vi "Exec-tempalate-test.vi"() -> ()   [LabVIEW 2021]
uses:
  Controls/Command_cluster.ctl
  Controls/Command_Enum.ctl
panel:
  in  "file (use dialog)":path
  out "index of element":i32
  out "Command":string
  in  "stop":bool
  out "1D Array":T1[](array[typedef])
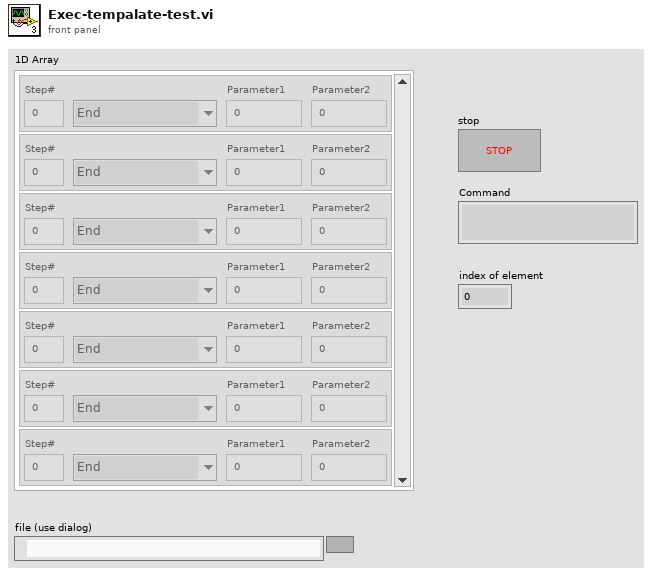
[diagram p1: front panel]
types:
  T1 = typedef "Command_cluster.ctl" = cluster{"Step#":dbl, "Commands":T2, "Parameter1":dbl, "Parameter2":dbl}
  T2 = typedef "Command_Enum.ctl" = enum16{"End", "Home All", "X Home", "Y Home", "X Move Rel", "X Move Abs", "Y Move Rel", "Y Move Abs", "Repeat", "Go To"}
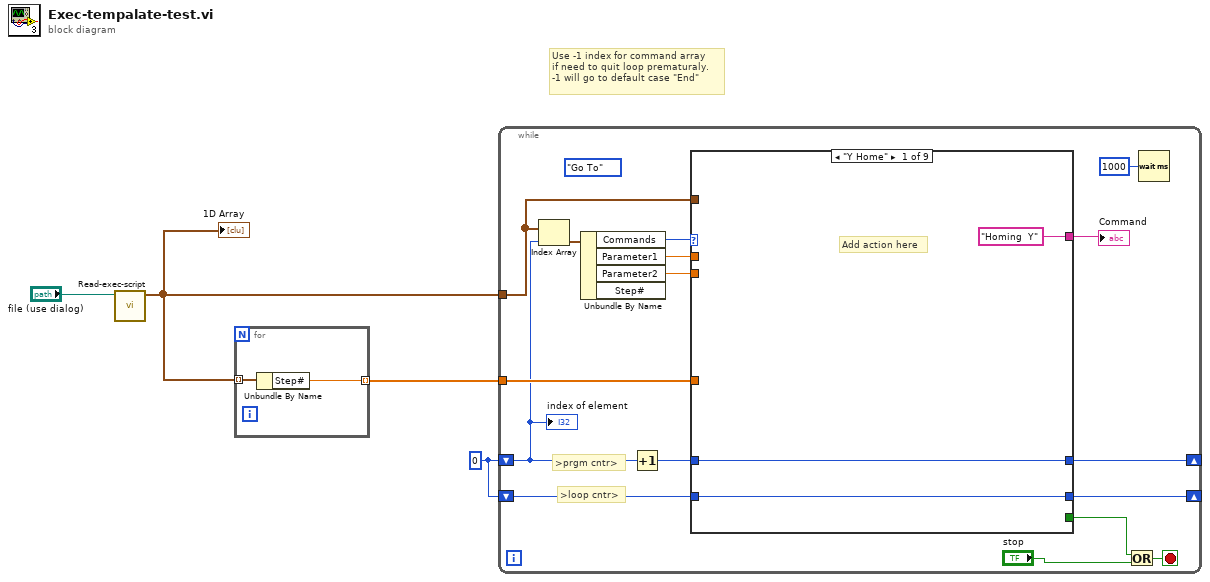
[diagram p0: block diagram]
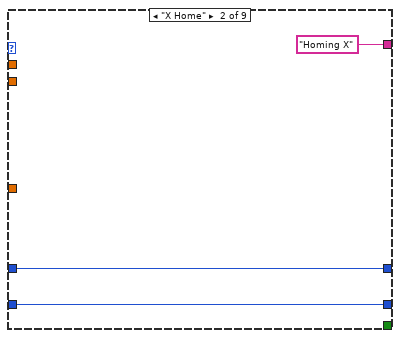
[diagram p2: hidden frame]
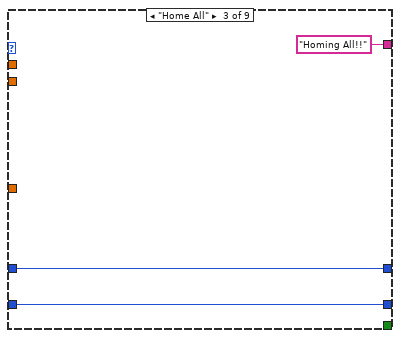
[diagram p3: hidden frame]
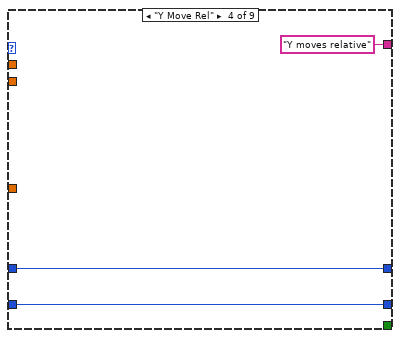
[diagram p4: hidden frame]
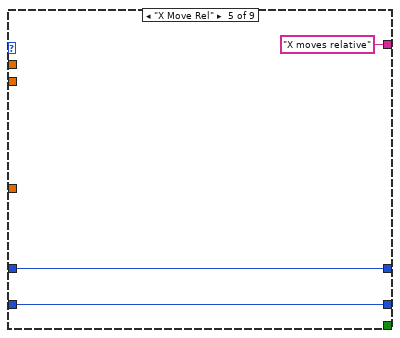
[diagram p5: hidden frame]
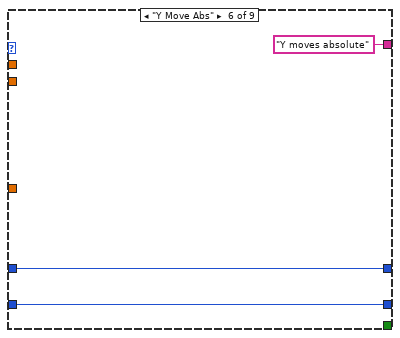
[diagram p6: hidden frame]
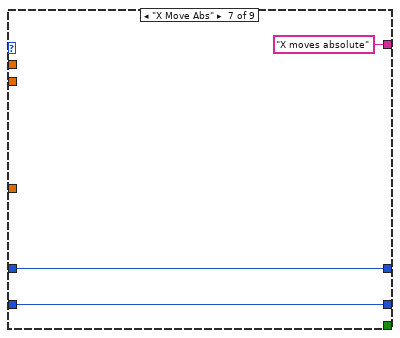
[diagram p7: hidden frame]
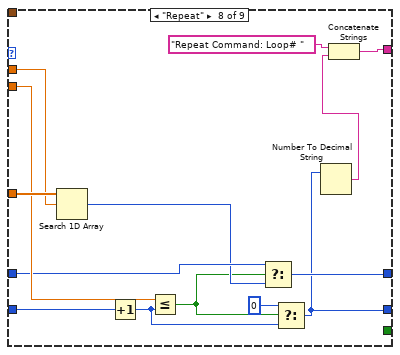
[diagram p8: hidden frame]
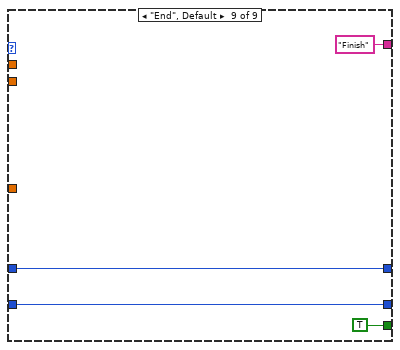
[diagram p9: hidden frame]
diagram:
  w3 = 0
  # "Use -1 index for command array\nif need to quit loop prematuraly.\n-1 will go to default case \"End\""
  n1 = call "Read-exec-script.vi"("file (use dialog)"="file (use dialog)") -> ("Commands"=w2:T1[])  [unwired: 9 in, 1 out]
  "1D Array" <- w2
  n2 = for {
    tunnel: w2 -> [w6] mode=indexing
    tunnel: [w5] -> w4 mode=indexing
    n3 = Unbundle By Name(w6) -> ("Step#"=w5:dbl)
  }
  n4 = while {
    tunnel: w2 -> [w17]
    tunnel: w4 -> [w18]
    shift-right: [w15] -> _
    shift-left: w3 -> [w8]
    shift-right: [w12] -> _
    shift-left: w3 -> [w16]
    stop <- w11 stop-if-true
    (unwired) Command_Enum."Go To" ("Commands")
    # ">loop cntr>"
    # ">prgm cntr>"
    n5 = Index Array(array=w17, index=w8) -> (element=w21:T1)
    n6 = Unbundle By Name(w21) -> ("Commands"=w7:T2, "Parameter1"=w19:dbl, "Parameter2"=w14:dbl)  [unwired: 1 out]
    n7 = Increment(x=w8) -> (x+1=w13:i32)
    n8 = case shown="\"Y Home\"" w7 {
      tunnel: ["Homing  Y" "Homing X" "Homing All!!" "Y moves relative" "X moves relative" "Y moves absolute" "X moves absolute" w44 "Finish"] -> w20
      tunnel: w19 -> [_ _ _ _ _ _ _ w56 _]
      tunnel: w18 -> [_ _ _ _ _ _ _ w57 _]
      tunnel: w17 -> [_ _ _ _ _ _ _ _ _]
      tunnel: w16 -> [w23 w26 w30 w32 w35 w38 w41 w55 w61]
      tunnel: [w24 w27 w29 w33 w36 w39 w42 w51 w60] -> w15
      tunnel: w14 -> [_ _ _ _ _ _ _ w54 _]
      tunnel: w13 -> [w24 w27 w29 w33 w36 w39 w42 w53 w60]
      tunnel: [w23 w26 w30 w32 w35 w38 w41 w46 w61] -> w12
      tunnel: [_ _ _ _ _ _ _ _ TRUE] -> w9
      frame "Y Home" {
        # "Add action here"
      }
      frame "X Home" {
      }
      frame "Home All" {
      }
      frame "Y Move Rel" {
      }
      frame "X Move Rel" {
      }
      frame "Y Move Abs" {
      }
      frame "X Move Abs" {
      }
      frame "Repeat" {
        n9 = Search 1D Array(1D array=w57, element=w56) -> (index of element=w52:i32)  [unwired: 1 in]
        n10 = Increment(x=w55) -> (x+1=w49:i32)
        n11 = Less Or Equal?(x=w54, y=w49) -> (x <= y?=w50:bool)
        n12 = Select(t=w53, s=w50, f=w52) -> (s? t:f=w51:i32)
        n13 = Select(t=0, s=w50, f=w49) -> (s? t:f=w46:i32)
        n14 = Number To Decimal String(number=w46) -> (decimal integer string=w45:string)  [unwired: 1 in]
        n15 = Concatenate Strings("Repeat Command: Loop# ", w45) -> (w44:string)
      }
      frame "End", Default {
      }
    }
    "Command" <- w20
    n16 = Or(x=w9, y="stop") -> (x .or. y?=w11:bool)
    n17 = Wait (ms)(milliseconds to wait=u32 1000) -> ()  [unwired: 1 out]
    "index of element" <- w8
  }
